vi "Word Easy Title.vi"(0 "report in":refnum<class "NI_report.lvclass">, 1 "font settings source":u16(ring) items=["VI Inputs", "Font Dialog Box"], 5 "title":string, 9 "font":T1={"font name"="", "font size"=18.0, "bold"=1, "italic"=0, "underline"=0, "strike through"=0, "font color"=16777216} {"font size" format="%0.2f"; "strike through" items=["Unchanged", "Yes", "No"]; "underline" items=["Unchanged", "Yes", "No"]; "italic" items=["Unchanged", "Yes", "No"]; "bold" items=["Unchanged", "Yes", "No"]}, 11 "error in (no error)":errorcluster) -> (4 "report out":refnum<class "NI_report.lvclass">, 6 "font out":T1={"font name"="", "font size"=0.0, "bold"=0, "italic"=0, "underline"=0, "strike through"=0, "font color"=16777216} {"font size" format="%0.2f"; "strike through" items=["Unchanged", "Yes", "No"]; "underline" items=["Unchanged", "Yes", "No"]; "italic" items=["Unchanged", "Yes", "No"]; "bold" items=["Unchanged", "Yes", "No"]}, 15 "error out":errorcluster)   [LabVIEW 2020, in "NI_ReportGenerationToolkit.lvlib"]
doc: "Adds a title to a Microsoft Word report."
uses:
  <vilib>/addons/_office/NI_ReportGenerationToolkit.lvlib
  <vilib>/Utility/NIReport.llb/NI_report.lvclass
  <vilib>/addons/_office/_exclsub.llb/font.ctl
  <vilib>/Utility/NIReport.llb/Append Report Text (str wrap).vi
  <vilib>/Utility/NIReport.llb/Word/NI_Word.lvclass
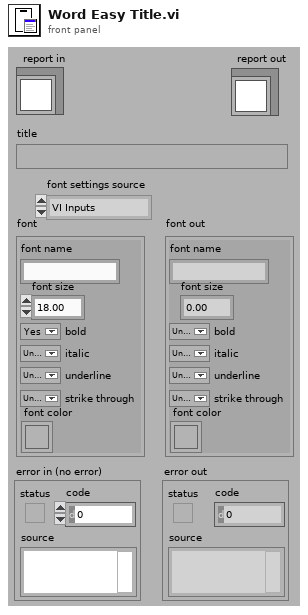
[diagram p1: front panel]
types:
  T1 = typedef "NI_ReportGenerationToolkit.lvlib/font.ctl" = cluster{"font name":string, "font size":dbl, "bold":u16, "italic":u16, "underline":u16, "strike through":u16, "font color":u32}
  T2 = cluster{"Charset (-1)":i16, "Weight (-1)":i16, "Name":string, "Size":string}
  T3 = cluster{i32, i32, i32, i32, "charset":i16, "weight":i16, "name":string, "size":string, "text color":u32}
  T4 = cluster{"italic":u16, "strike through":u16, "underline":u16, "bold":u16}
  T5 = typedef "NI_ReportGenerationCore.lvlib/font.ctl" = cluster{"font name":string, "font size":dbl, "bold":u16, "italic":u16, "underline":u16, "strike through":u16, "font color":u32}
  T6 = cluster{"Alignment":enum16{"Left", "Centered", "Right", "Justify"}, "Left":dbl, "Right":dbl, "Special":enum16{"(none)", "First line", "Hanging"}, "By":dbl, "Before":dbl, "After":dbl, "Line spacing":enum16{"Single", "1,5 lines", "Double", "At least", "Exactly", "Multiple"}, "At":dbl}
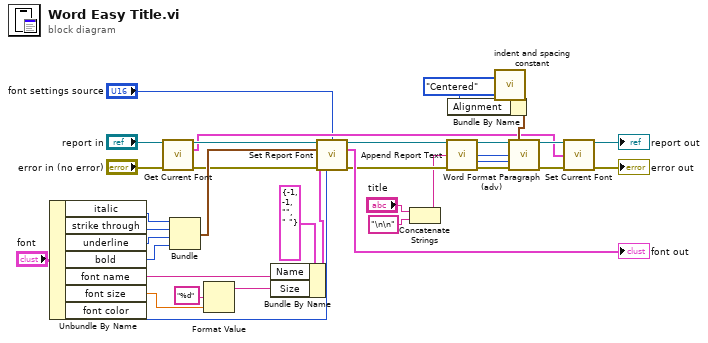
[diagram p0: block diagram]
diagram:
  n1 = Unbundle By Name("font") -> ("italic"=w23:u16, "strike through"=w26:u16, "underline"=w25:u16, "bold"=w24:u16, "font name"=w28:string, "font size"=w30:dbl, "font color"=w21:u32)
  n2 = call <vilib>:"Get Current Font.vi"("report in"="report in", "error in (no error)"="error in (no error)") -> ("report.lvclass"=w15:refnum<class "NI_report.lvclass">, "font"=w10:T3, "error out"=w16:errorcluster)  [unwired: 11 out]
  n3 = Bundle("italic"=w23, "strike through"=w26, "underline"=w25, "bold"=w24) -> (w22:T4)  [unwired: 1 out]
  n4 = Format Value(format string="%d", value (0)=w30) -> (output string=w27:string)  [unwired: 1 out]
  n5 = Bundle By Name(cluster=T2 {"Charset (-1)"=-1, "Weight (-1)"=-1, "Name"="", "Size"=" "} ("font settings"), "Name"=w28, "Size"=w27) -> (w36:T2)
  n6 = call-dynamic "Set Report Font.vi"("report in"=w15, "text color (unchanged)"=w21, "font settings source (VI Inputs)"="font settings source", "text options"=w22, "font settings"=w36, "error in (no error)"=w16) -> ("report out"=w7:refnum<class "NI_report.lvclass">, "font out"=→"font out":T5, "error out"=w6:errorcluster)  [unwired: 7 in]
  n7 = Concatenate Strings("title", "\n\n" ("Substring")) -> (w5:string)
  n8 = call-poly <vilib>:"Append Report Text.vi"("report in"=w7, "text"=w5, "error in (no error)"=w6) -> ("report out"=w4:refnum<class "NI_report.lvclass">, "start out (Word)"=w2:i32, "end out (Word)"=w1:i32, "error out"=w3:errorcluster)  [unwired: 3 in, 6 out]
  n9 = call <vilib>:"indent and spacing constant.vi"() -> ("indent and spacing"=w32:T6)
  n10 = Bundle By Name(cluster=w32, "Alignment"=enum16{"Left", "Centered", "Right", "Justify"}."Centered") -> (w33:T6)
  n11 = call <vilib>:"Word Format Paragraph (adv).vi"("report in"=w4, "indent and spacing"=w33, "start (-1)"=w2, "end (-1)"=w1, "error in (no error)"=w3) -> ("report out"=w13:refnum<class "NI_report.lvclass">, "error out"=w14:errorcluster)  [unwired: 2 in, 7 out]
  n12 = call <vilib>:"Set Current Font.vi"("report in"=w13, "font"=w10, "error in (no error)"=w14) -> ("report out"=→"report out":refnum<class "NI_report.lvclass">, "error out"=→"error out":errorcluster)  [unwired: 11 out]
